vi "CollideDriveX.vi"(10 "Setpoint":dbl, 11 "Setpoint":dbl) -> ()   [LabVIEW 2017]
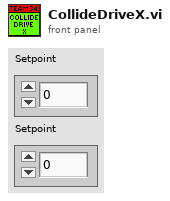
[diagram p1: front panel]
types:
  T1 = typedef "WPI_AccelerometerDevRef.ctl" = cluster{"DevStatus":errorcluster, "Scaling":T2, "Analog Channels":T3, "I2C Bus":T5, "SPI Bus":T6, "Accel Range":T7, "ADXL Axes":T8, "Handle":i32, "Device Address":u8, "Accel Type":enum16{"Analog", "ADXL345 I2C", "ADXL345 SPI", "Internal", "ADXL362 SPI"}}
  T2 = typedef "WPI_AccelerometerScaling.ctl" = cluster{"Gain (VoltsPerG)":dbl, "Center Voltage":dbl}
  T3 = typedef "WPI_AccelerometerAnalogChannels.ctl" = cluster{"X-Axis":T4, "Y-Axis":T4, "Z-Axis":T4}
  T4 = typedef "FPGA_AIChannel.ctl" = enum8{"AI 0", "AI 1", "AI 2", "AI 3", "AI MXP 0", "AI MXP 1", "AI MXP 2", "AI MXP 3", "Invalid"}
  T5 = typedef "i2c_bus.ctl" = enum16{"I2C On-Board", "I2C MXP", "Invalid"}
  T6 = typedef "spi_bus.ctl" = enum16{"SPI On-Board, CS0", "SPI On-Board, CS1", "SPI On-Board, CS2", "SPI On-Board, CS3", "SPI MXP", "Invalid"}
  T7 = typedef "ADXL345 Range.ctl" = u8
  T8 = typedef "WPI_AccelerometerADXL345 Axes.ctl" = cluster{"X-Axis":bool, "Y-Axis":bool, "Z-Axis":bool}
  T9 = cluster{"X-Axis":dbl, "Y-Axis":dbl, "Z-Axis":dbl}
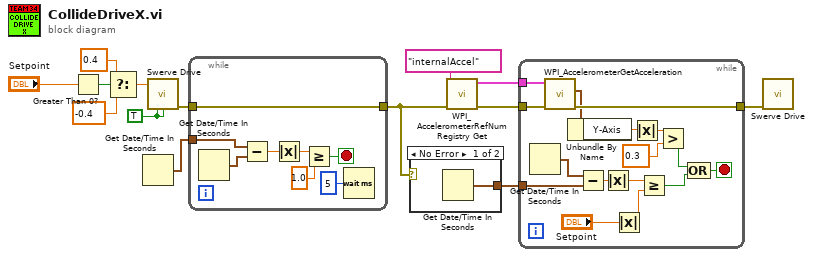
[diagram p0: block diagram]
diagram:
  w5 = TRUE ("Robot Centric?")
  n1 = Greater Than 0?(x="Setpoint") -> (x > 0?=w1:bool)
  n2 = Select(t=0.4, s=w1, f=-0.4) -> (s? t:f=w4:dbl)
  n3 = Get Date/Time In Seconds() -> (seconds since 1Jan1904=w8:timestamp)
  n4 = call "Swerve Drive.vi"("X"=w4, "Robot Centric?"=w5, "Autonomous?"=w5) -> ("Error Out"=w6:errorcluster)  [unwired: 8 in, 4 out]
  n5 = while {
    tunnel: w6 -> [w22]
    tunnel: [w22] -> w9
    tunnel: w8 -> [w21]
    stop <- w16 stop-if-true
    n6 = Get Date/Time In Seconds() -> (seconds since 1Jan1904=w20:timestamp)
    n7 = Subtract(x=w21, y=w20) -> (x-y=w19:dbl)
    n8 = Absolute Value(x=w19) -> (abs(x)=w18:dbl)
    n9 = Greater Or Equal?(x=w18, y=1.0) -> (x >= y?=w16:bool)
    n10 = Wait (ms)(milliseconds to wait=u32 5) -> ()  [unwired: 1 out]
  }
  n11 = case shown="No Error" w9 {
    tunnel: [w23 _] -> w7
    frame No Error {
      n12 = Get Date/Time In Seconds() -> (seconds since 1Jan1904=w23:timestamp)
    }
    frame Error {
    }
  }
  n13 = call <vilib>:"WPI_AccelerometerRefNum Registry Get.vi"("error in (no error)"=w9, "refnum name"="internalAccel") -> ("error out"=w12:errorcluster, "AccelerometerDevRef"=w11:T1)  [unwired: 8 in]
  n14 = while {
    tunnel: w7 -> [w36]
    tunnel: w11 -> [w39]
    tunnel: w12 -> [w38]
    tunnel: [w32] -> w13
    stop <- w25 stop-if-true
    n15 = Get Date/Time In Seconds() -> (seconds since 1Jan1904=w37:timestamp)
    n16 = call <vilib>:"WPI_AccelerometerGetAcceleration.vi"("error in"=w38, "AccelerometerDevRef"=w39) -> ("error out"=w32:errorcluster, "Accelerations"=w31:T9)  [unwired: 7 in, 1 out]
    n17 = Unbundle By Name(w31) -> ("Y-Axis"=w30:dbl)
    n18 = Subtract(x=w37, y=w36) -> (x-y=w35:dbl)
    n19 = Absolute Value(x=w35) -> (abs(x)=w34:dbl)
    n20 = Absolute Value(x="Setpoint") -> (abs(x)=w33:dbl)
    n21 = Absolute Value(x=w30) -> (abs(x)=w29:dbl)
    n22 = Greater Or Equal?(x=w34, y=w33) -> (x >= y?=w26:bool)
    n23 = Greater?(x=w29, y=0.3) -> (0:w27:bool)
    n24 = Compound Arithmetic op=OR(w27, w26) -> (w25:bool)
  }
  n25 = call "Swerve Drive.vi"("Error In"=w13) -> ()  [unwired: 10 in, 5 out]
